vi "Step_Delay_Tommaso_equal_output.vi"() -> ()   [LabVIEW 2015]
uses:
  <vilib>/DAQmx/write.llb/DAQmx Write (Analog DBL 1Chan 1Samp).vi
  <vilib>/DAQmx/miscellaneous.llb/DAQmx Fill In Error Info.vi
  <vilib>/DAQmx/create/channels.llb/DAQmx Create Channel (AO-Voltage-Basic).vi
  <vilib>/Analysis/1siggen.llb/Ramp Pattern by Delta.vi
  subvi/Newport ESP301/Newport ESP301.lvlib
  <vilib>/Analysis/NI_AALBase.lvlib
panel:
  in  "Output_Steps":bool caption="Output steps?"
  in  "Dwell_positions":string[][](table)=[["-500", "3000"], ["-100", "3000"], ["0", "5000"], ["100", "5000"], ["500", "5000"], ["750", "10000"], ["1000", "10000"], ["", ""]]
  in  "Enable2":bool caption="Enable?"
  in  "Wait time [ms]":u32=1000 caption="Values <50 \nwon't work"
  out "StepSize [mm]":dbl=0.14989622900000002
  in  "stop 2":bool
  in  "StepSize [fs]":i32=1000
  in  "Enable?":bool
  out "a":waveform(dbl)(graph)={"t0"=timestamp(3629703941.150015 s since 1904-01-01), "dt"=1.0, "Y"=[-1.00695]}
  out "Waveform Chart":dbl(graph)=5.25341140860948
  out "x*y":dbl=0.9998993703837595
  in  "physical channels":tag="Dev3/ao1"
  out "DAC error":errorcluster
  out "ESP error":errorcluster
  out "run?":bool
  in  "set_vel":bool
  in  "velocity [fs/s]":dbl=333.564095198152
  in  "vel_mm":dbl=0.05 caption="velocity [mm/s]"
  out "meas. velocity":dbl
  in  "stop":bool
  out "output voltage":dbl=0.9998993703837595
  in  "start":bool
  in  "go2p1":bool
  out "position [mm]":dbl=-1.00695
  in  "p2 [mm]":dbl=-0.707153771
  in  "p1 [mm]":dbl=-1.006946229
  in  "interpolate output":bool
  in  "Delta2 [fs]":dbl=999.9999999999999
  in  "Delta1 [fs]":dbl=-999.9999999999999
  in  "Reference [mm]":dbl=-0.85705
  in  "Axis (1)":i32=3 min=1 max=3
  in  "Serial Link (RS232)":enum16{"RS232", "USB"}(ring)
  in  "VISA resource name":refnum<visa-resource-name>="COM9"
  in  "main_close":bool
  # "Interface panel"
  # "Velocity panel"
  # "Positions panel"
  # "Equally spaced steps panel"
  # "Controls panel"
  # "User-defined steps panel"
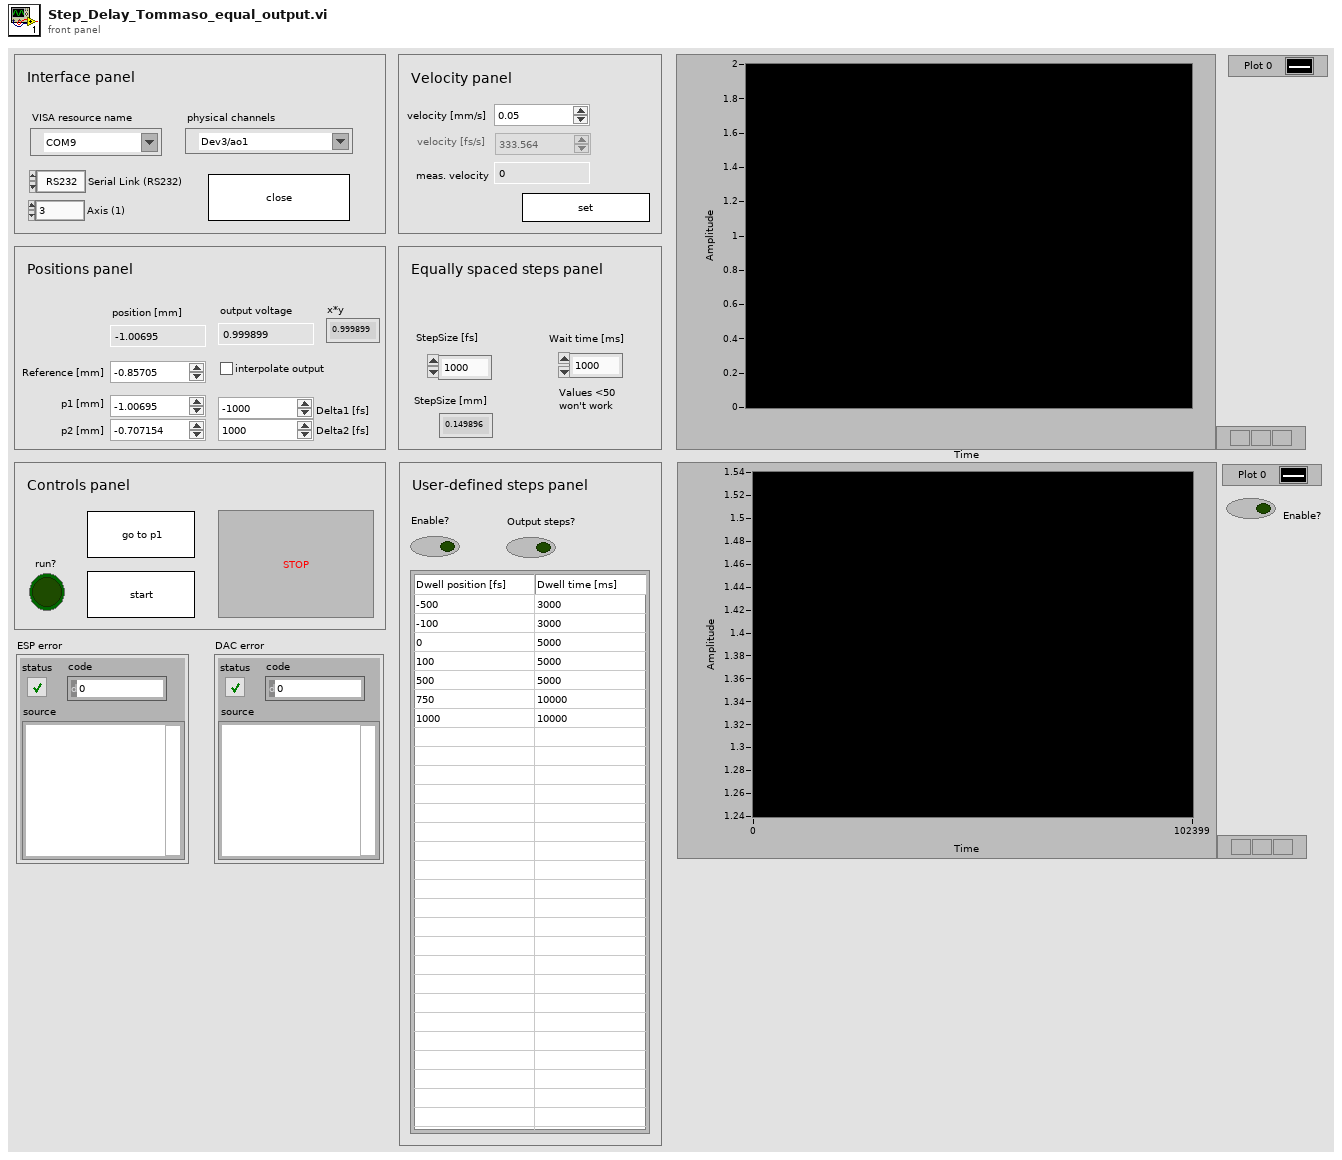
[diagram p1: front panel]
types:
  T1 = cluster{"dev1_data":refnum<queue>, "dev2_data":refnum<queue>}
  T2 = cluster{"dev1_cmd":refnum<queue>, "dev2_cmd":refnum<queue>}
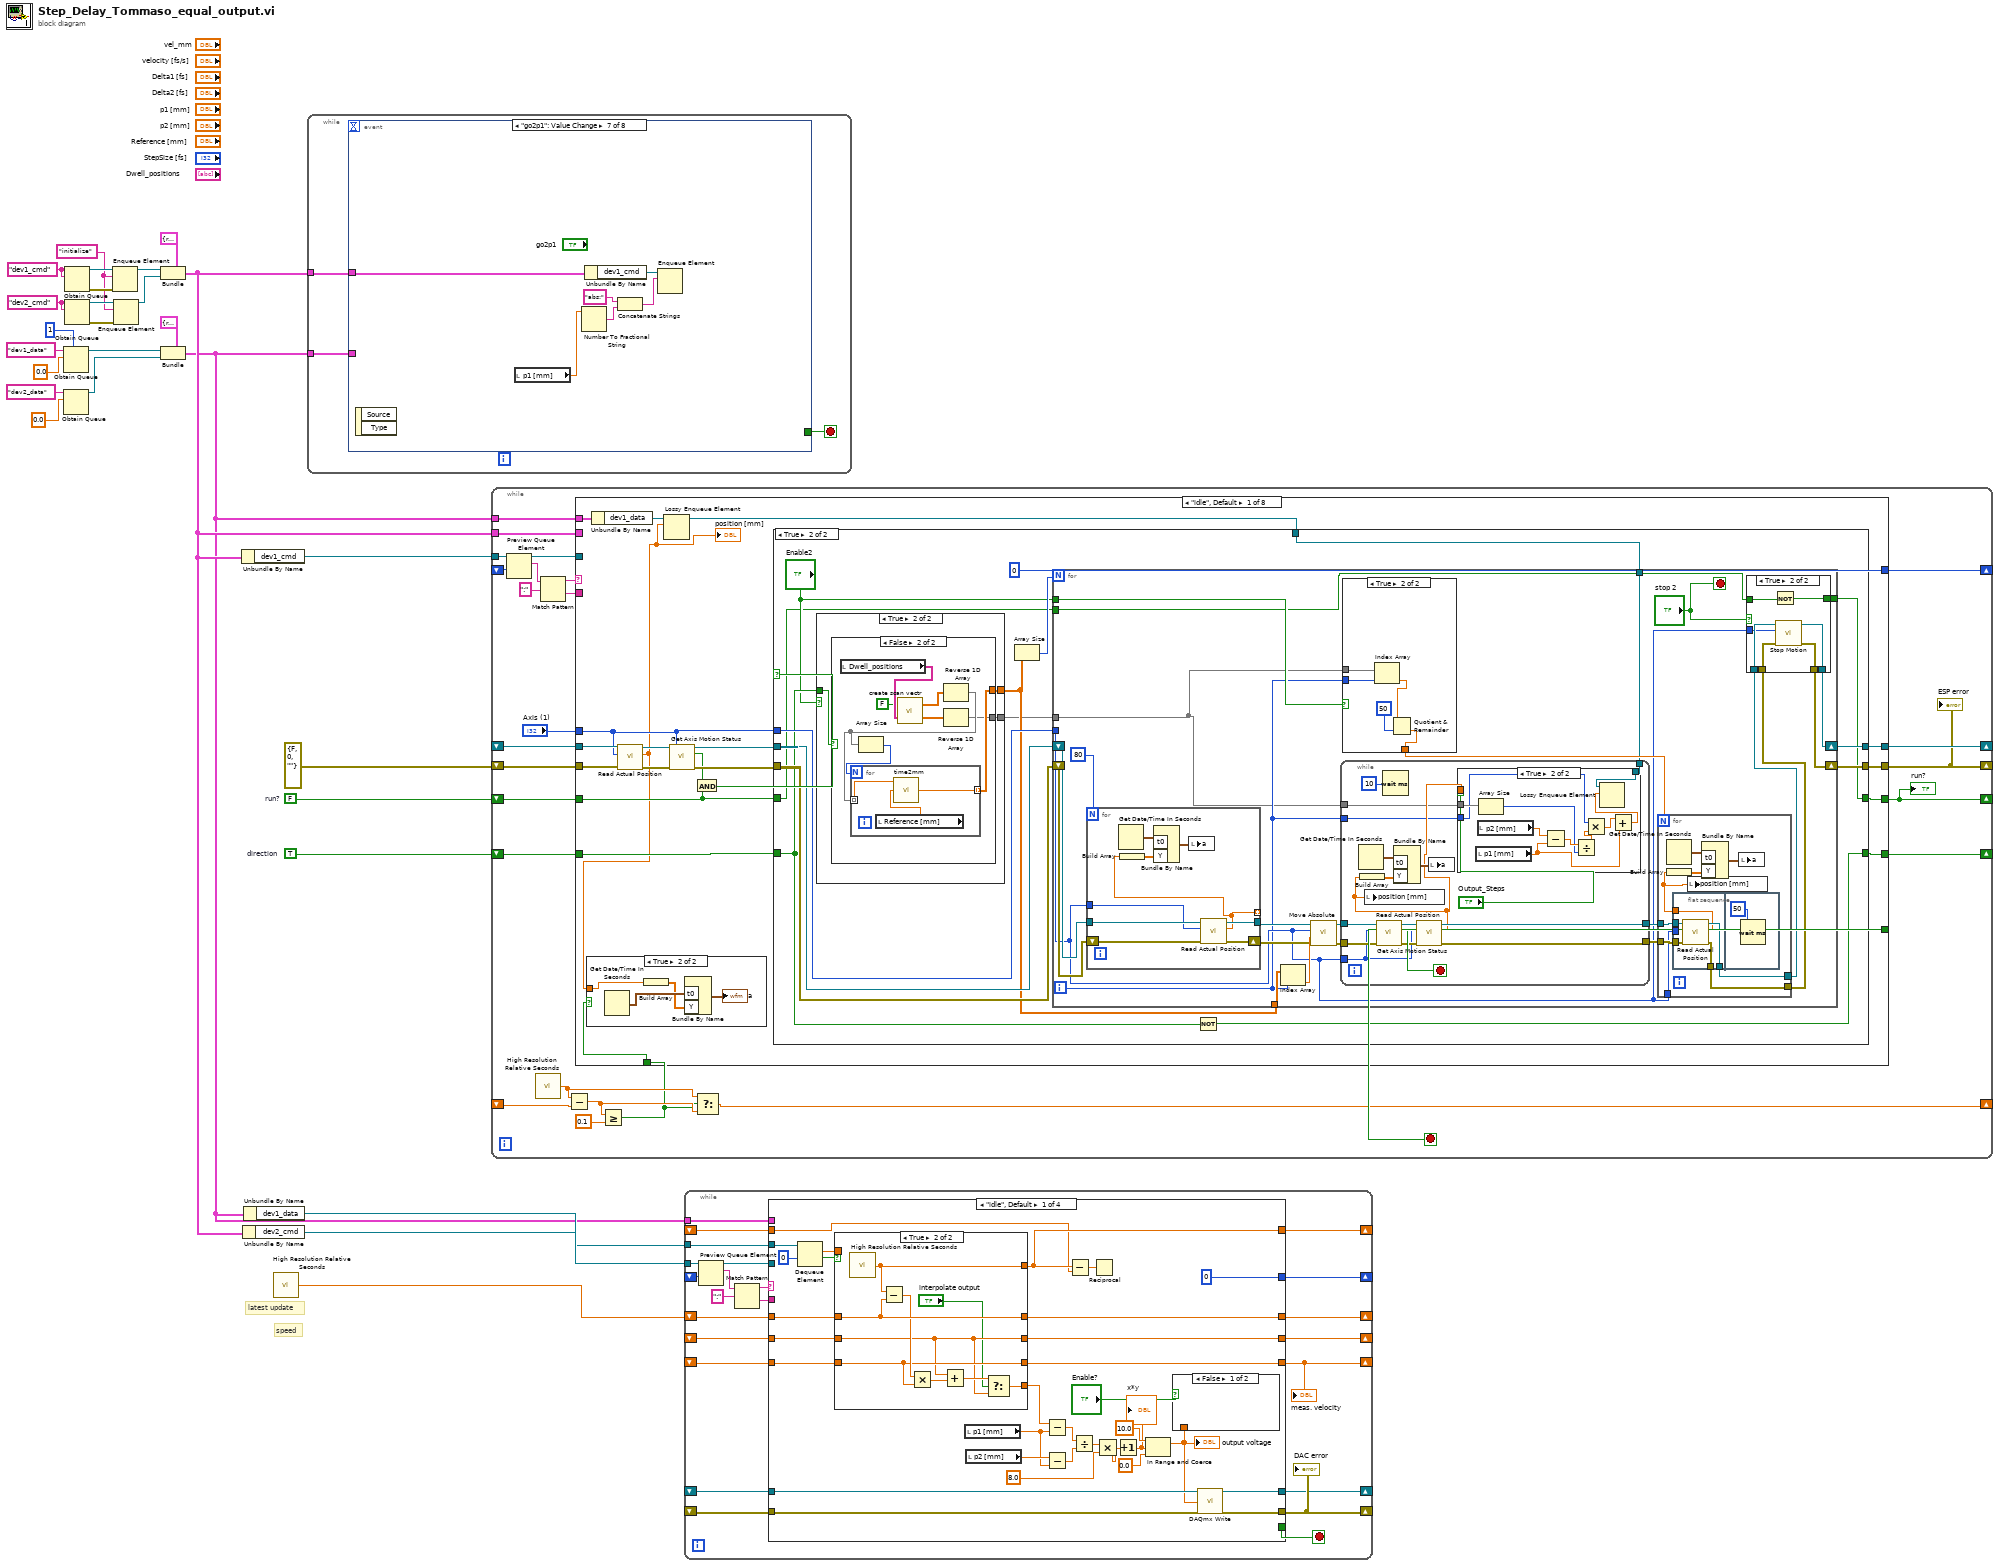
[diagram p0: block diagram]
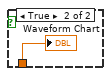
[diagram p2: hidden frame]
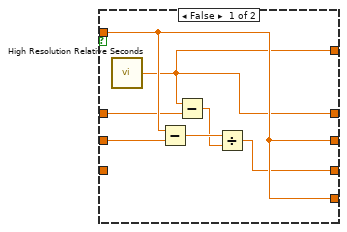
[diagram p3: hidden frame]
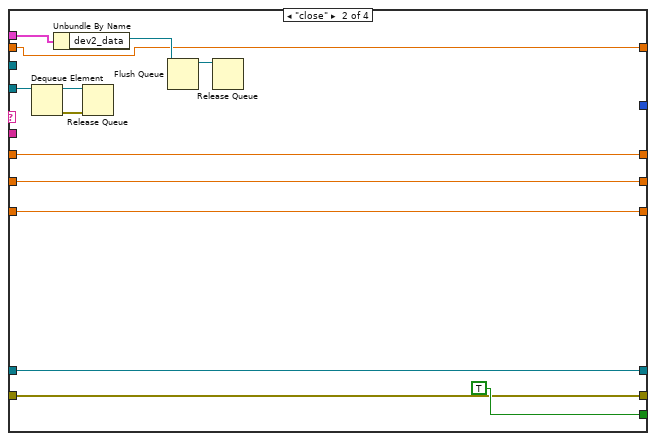
[diagram p4: hidden frame]
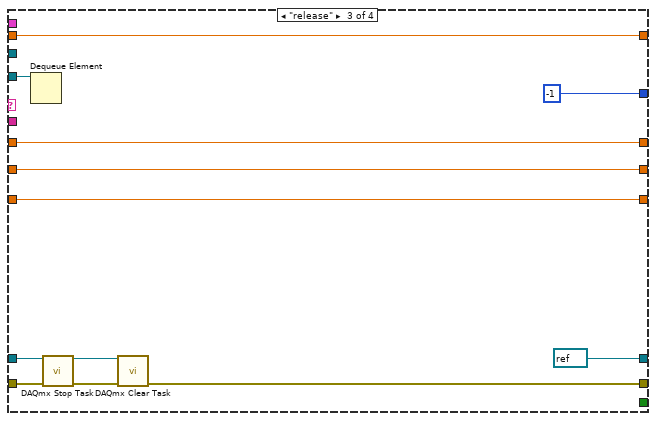
[diagram p5: hidden frame]
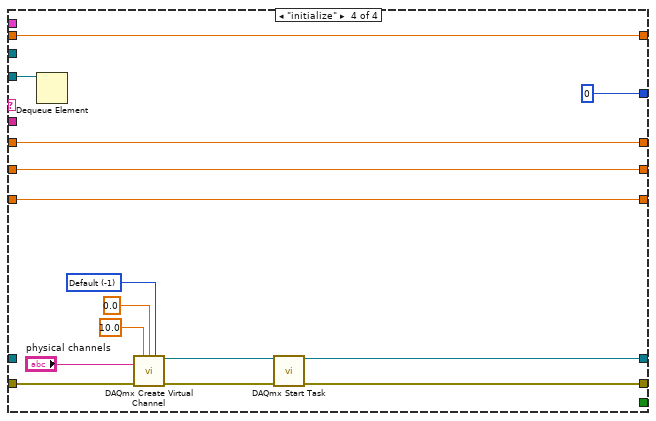
[diagram p6: hidden frame]
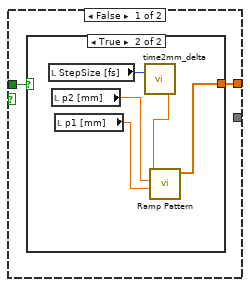
[diagram p9: hidden frame]
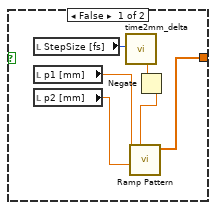
[diagram p10: hidden frame]
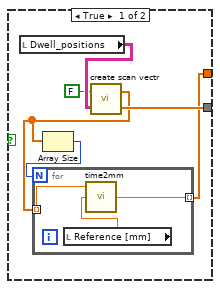
[diagram p11: hidden frame]
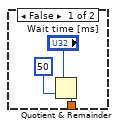
[diagram p13: hidden frame]
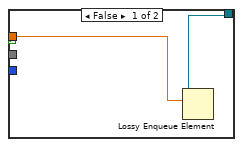
[diagram p14: hidden frame]
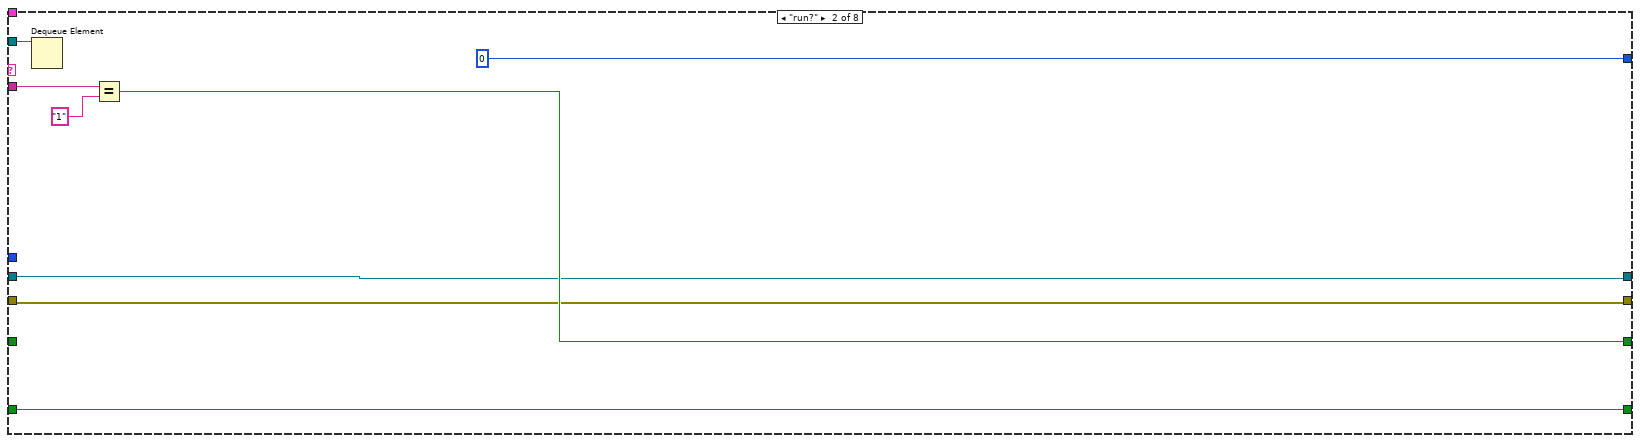
[diagram p15: hidden frame]
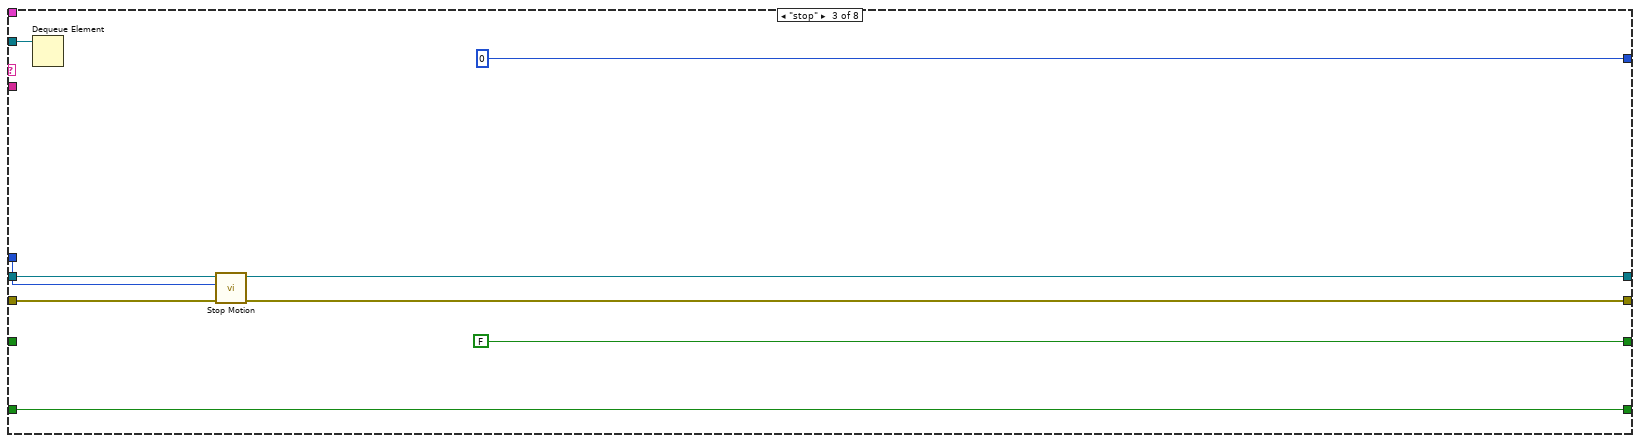
[diagram p16: hidden frame]
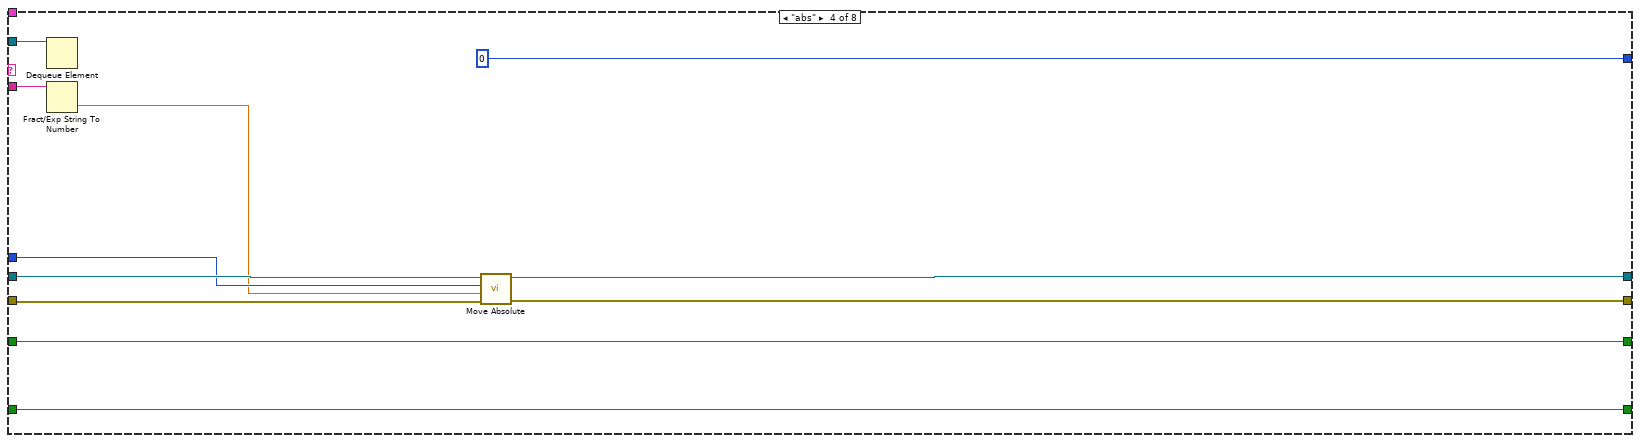
[diagram p17: hidden frame]
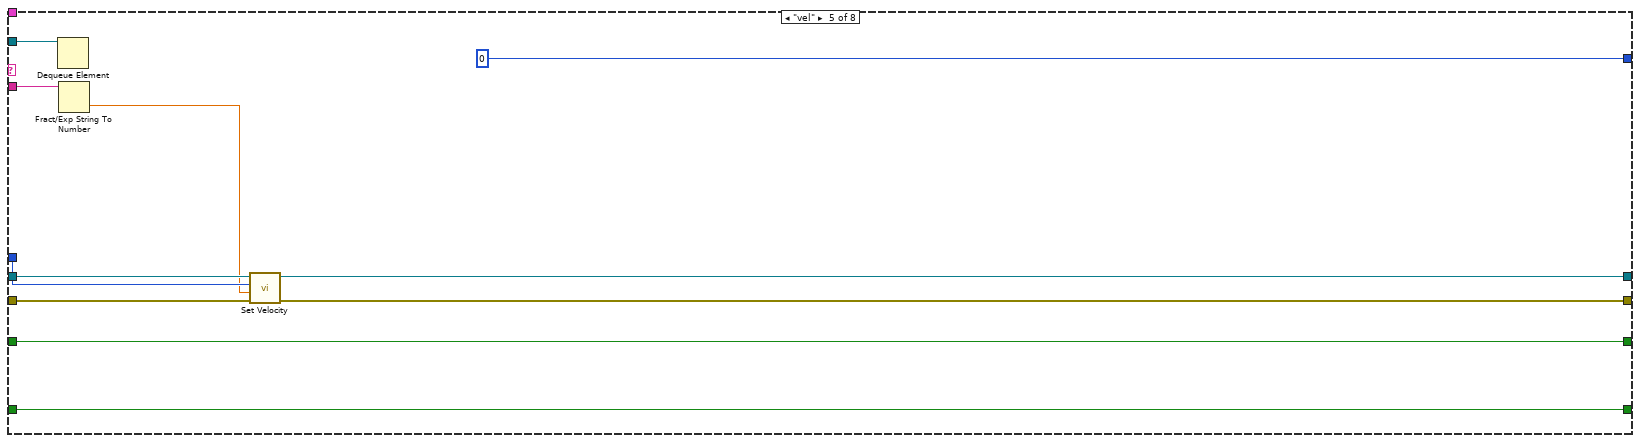
[diagram p18: hidden frame]
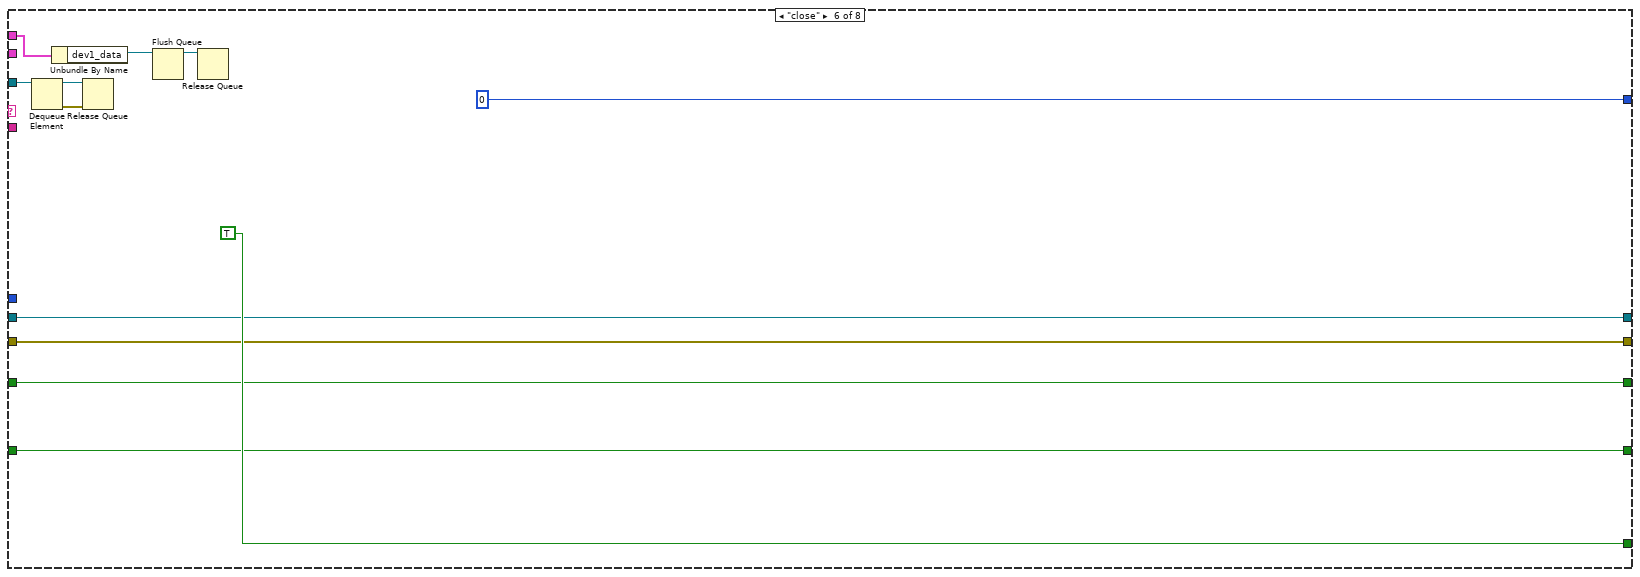
[diagram p19: hidden frame]
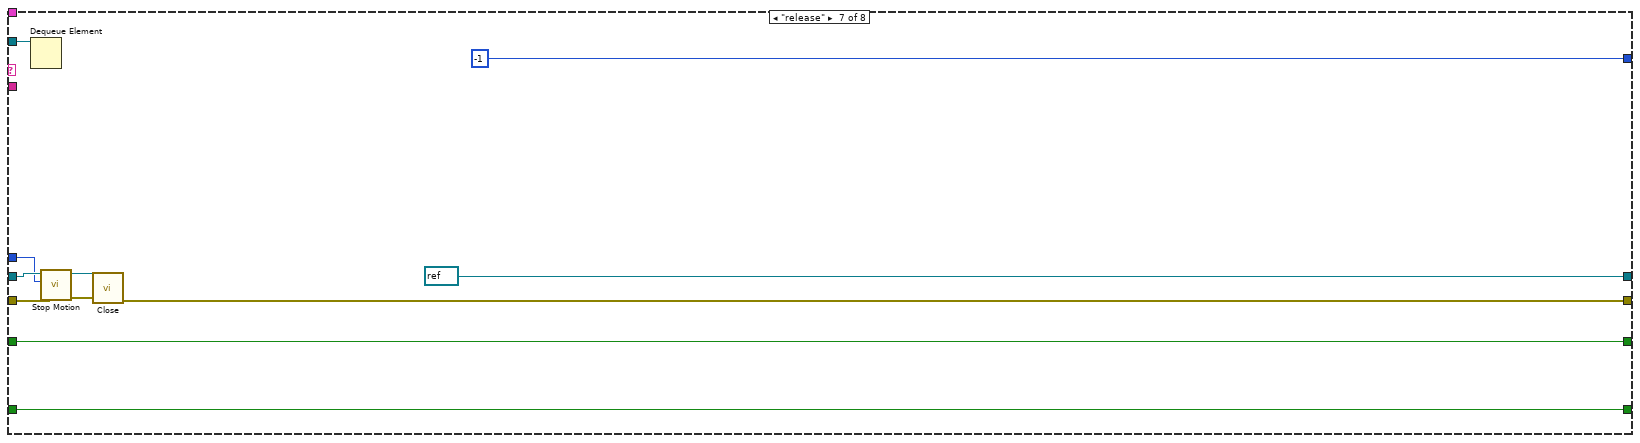
[diagram p20: hidden frame]
diagram:
  w1 = TRUE  # direction
  w4 = FALSE  # run?
  w15 = "dev2_cmd" ("name (unnamed)")
  w21 = "initialize" ("element")
  w16 = "dev1_cmd" ("name (unnamed)")
  # "speed"
  # "latest update"
  n1 = Obtain Queue(max queue size (-1, unlimited)=1, name (unnamed)="dev1_data", element data type=0.0) -> (queue out=w12:refnum<queue>)  [unwired: 2 in, 2 out]
  n2 = Obtain Queue(name (unnamed)="dev2_data", element data type=0.0) -> (queue out=w11:refnum<queue>)  [unwired: 3 in, 2 out]
  n3 = Obtain Queue(name (unnamed)=w16, element data type=w16) -> (queue out=w27:refnum<queue>, error out=w26:errorcluster)  [unwired: 3 in, 1 out]
  n4 = Obtain Queue(name (unnamed)=w15, element data type=w15) -> (queue out=w22:refnum<queue>, error out=w23:errorcluster)  [unwired: 3 in, 1 out]
  n5 = Enqueue Element(queue=w27, element=w21, error in (no error)=w26) -> (queue out=w24:refnum<queue>)  [unwired: 1 in, 2 out]
  n6 = Enqueue Element(queue=w22, element=w21, error in (no error)=w23) -> (queue out=w20:refnum<queue>)  [unwired: 1 in, 2 out]
  n7 = Bundle(cluster=T2 {"dev1_cmd"=refnum, "dev2_cmd"=refnum}, "dev1_cmd"=w24, "dev2_cmd"=w20) -> (w8:T2)
  n8 = Bundle(cluster=T1 {"dev1_data"=refnum, "dev2_data"=refnum}, "dev1_data"=w12, "dev2_data"=w11) -> (w2:T1)
  n9 = Unbundle By Name(w8) -> ("dev1_cmd"=w17:refnum<queue>)
  n10 = Unbundle By Name(w8) -> ("dev2_cmd"=w7:refnum<queue>)
  n11 = Unbundle By Name(w2) -> ("dev1_data"=w6:refnum<queue>)
  n12 = call <vilib>:"High Resolution Relative Seconds.vi"() -> ("relative seconds"=w5:dbl)
  n13 = while {
    tunnel: w8 -> [w30]
    tunnel: w2 -> [w29]
    stop <- w28 stop-if-true
    n14 = event shown="[6] \"go2p1\": Value Change" {
      selector: _ -> [_ _ _ _ _ _ _ _]
      dyn-events: _ -> [_ _ _ _ _ _ _ _]
      timeout: _ -> [_ _ _ _ _ _ _ _]
      tunnel: w30 -> [_ w34 _ _ w46 _ w64 w67]
      tunnel: w29 -> [_ _ _ _ _ _ _ _]
      tunnel: [_ _ _ _ _ _ _ TRUE] -> w28
      event Timeout {
        n15 = event-data() -> ()  [unwired: 1 in, 1 out]
      }
      event "start", "stop": Value Change {
        n16 = event-data() -> ()  [unwired: 1 in, 1 out]
        n17 = Boolean To (0,1)(Boolean="start") -> (0, 1=w32:i16)
        n18 = Number To Decimal String(number=w32) -> (decimal integer string=w31:string)  [unwired: 1 in]
        n19 = Unbundle By Name(w34) -> ("dev1_cmd"=w37:refnum<queue>)
        n20 = Concatenate Strings("run?:" ("string"), w31) -> (w36:string)
        n21 = Enqueue Element(queue=w37, element=w36) -> ()  [unwired: 2 in, 3 out]
      }
      event "StepSize [fs]": Value Change {
        n22 = event-data() -> ("NewVal"=w38:i32)  [unwired: 1 in, 5 out]
        n23 = call "time2mm_delta.vi"("Delta time"=w38) -> ("Delta position (mm)"=→"StepSize [mm]":dbl)  [unwired: 2 in]
      }
      event "Delta1 [fs]", "Delta2 [fs]": Value Change {
        n24 = event-data() -> ()  [unwired: 1 in, 1 out]
        n25 = local read "Reference [mm]"() -> (w41:dbl)
        n26 = local read "Delta2 [fs]"() -> (w42:dbl)
        n27 = local read "Delta1 [fs]"() -> (w44:dbl)
        n28 = call "time2mm.vi"("Offset (mm)"=w41, "time"=w44) -> ("position (mm)"=w43:dbl)  [unwired: 1 in]
        n29 = call "time2mm.vi"("Offset (mm)"=w41, "time"=w42) -> ("position (mm)"=w40:dbl)  [unwired: 1 in]
        n30 = local write "p2 [mm]"(w40) -> ()
        n31 = local write "p1 [mm]"(w43) -> ()
      }
      event "set_vel": Value Change {
        n32 = event-data() -> ()  [unwired: 1 in, 2 out]
        n33 = local read "vel_mm"() -> (w45:dbl)
        n34 = Number To Fractional String(number=w45) -> (F-format string=w49:string)  [unwired: 3 in]
        n35 = Unbundle By Name(w46) -> ("dev1_cmd"=w50:refnum<queue>)
        n36 = Concatenate Strings("vel:" ("string"), w49) -> (w48:string)
        n37 = Enqueue Element(queue=w50, element=w48) -> ()  [unwired: 2 in, 3 out]
      }
      event "p1 [mm]", "p2 [mm]", "Reference [mm]", "vel_mm": Value Change {
        n38 = event-data() -> ()  [unwired: 1 in, 2 out]
        n39 = local read "Reference [mm]"() -> (w56:dbl)
        n40 = local read "vel_mm"() -> (w53:dbl)
        n41 = local read "p1 [mm]"() -> (w57:dbl)
        n42 = local read "p2 [mm]"() -> (w58:dbl)
        n43 = call "mm2time.vi"("Offset (mm)"=0.0, "distance (mm)"=w53) -> ("time in fs"=w52:dbl)  [unwired: 1 in]
        n44 = call "mm2time.vi"("Offset (mm)"=w56, "distance (mm)"=w57) -> ("time in fs"=w54:dbl)  [unwired: 1 in]
        n45 = call "mm2time.vi"("Offset (mm)"=w56, "distance (mm)"=w58) -> ("time in fs"=w55:dbl)  [unwired: 1 in]
        n46 = local write "velocity [fs/s]"(w52) -> ()
        n47 = local write "Delta1 [fs]"(w54) -> ()
        n48 = local write "Delta2 [fs]"(w55) -> ()
      }
      event "go2p1": Value Change {
        n49 = event-data() -> ()  [unwired: 1 in, 2 out]
        n50 = local read "p1 [mm]"() -> (w59:dbl)
        n51 = Number To Fractional String(number=w59) -> (F-format string=w62:string)  [unwired: 3 in]
        n52 = Unbundle By Name(w64) -> ("dev1_cmd"=w63:refnum<queue>)
        n53 = Concatenate Strings("abs:" ("string"), w62) -> (w60:string)
        n54 = Enqueue Element(queue=w63, element=w60) -> ()  [unwired: 2 in, 3 out]
      }
      event "main_close": Value Change {
        n55 = event-data() -> ()  [unwired: 1 in, 1 out]
        n56 = Cluster To Array(cluster=w67) -> (array=w66:refnum<queue>[])
        n57 = for {
          tunnel: w66 -> [w72] mode=indexing
          n58 = Flush Queue(queue=w72) -> (queue out=w68:refnum<queue>)  [unwired: 1 in, 2 out]
          n59 = Enqueue Element(queue=w68, element="release") -> (queue out=w70:refnum<queue>)  [unwired: 2 in, 2 out]
          n60 = Enqueue Element(queue=w70, element="close") -> ()  [unwired: 2 in, 3 out]
        }
      }
    }
  }
  n61 = while {
    tunnel: w8 -> [w93]
    tunnel: w17 -> [w98]
    tunnel: w2 -> [w90]
    shift-right: [w88] -> _
    shift-left: _ -> [w89]
    shift-right: [w87] -> _
    shift-left: _ -> [w84]
    shift-right: [w86] -> _
    shift-left: errorcluster {"status"=FALSE, "code"=0, "source"=""} ("error out") -> [w85]
    shift-right: [w81] -> _
    shift-left: w4 -> [w82]
    shift-right: [w79] -> _
    shift-left: w1 -> [w80]
    shift-right: [w73] -> _
    shift-left: _ -> [w78]
    stop <- w91 stop-if-true
    n62 = Preview Queue Element(queue=w98, timeout in ms (-1)=w89) -> (queue out=w92:refnum<queue>, element=w97:string)  [unwired: 1 in, 2 out]
    n63 = call <vilib>:"High Resolution Relative Seconds.vi"() -> ("relative seconds"=w75:dbl)
    n64 = Match Pattern(string=w97, regular expression=":") -> (before substring=w95:string, after substring=w94:string)  [unwired: 1 in, 2 out]
    n65 = Subtract(x=w75, y=w78) -> (x-y=w76:dbl)
    n66 = Greater Or Equal?(x=w76, y=0.1) -> (x >= y?=w74:bool)
    n67 = case shown="\"idle\", Default" w95 {
      tunnel: w94 -> [_ w281 _ w300 w307 _ _ _]
      tunnel: w93 -> [_ _ _ _ _ _ _ _]
      tunnel: w92 -> [_ w279 w283 w301 w305 w324 w334 w344]
      tunnel: [_ _ _ _ _ TRUE _ _] -> w91
      tunnel: w90 -> [w118 _ _ _ _ w316 _ _]
      tunnel: [0 0 0 0 0 0 -1 0] -> w88
      tunnel: [w116 w274 w288 w297 w312 w320 refnum<visa-resource-name> refnum ("VISA resource name out") w340] -> w87
      tunnel: [w115 w275 w287 w296 w311 w319 w333 w339] -> w86
      tunnel: w85 -> [w113 w275 w289 w298 w310 w319 w329 _]
      tunnel: w84 -> [w114 w274 w290 w299 w309 w320 w326 _]
      tunnel: "Axis (1)" -> [w104 _ w286 w295 w308 _ w325 w341]
      tunnel: w82 -> [w102 _ _ w292 w303 w317 w331 w345]
      tunnel: [w110 w277 FALSE ("run?") w292 w303 w317 w331 w345] -> w81
      tunnel: w80 -> [w111 w276 w282 w291 w302 w313 w330 w336]
      tunnel: [w112 w276 w282 w291 w302 w313 w330 w336] -> w79
      tunnel: w74 -> [w99 _ _ _ _ _ _ _]
      frame "idle", Default {
        n68 = Unbundle By Name(w118) -> ("dev1_data"=w117:refnum<queue>)
        n69 = call "Read Actual Position.vi"("error in (no error)"=w113, "Axis (1)"=w104, "VISA resource name"=w114) -> ("error out"=w107:errorcluster, "Position (units)"=w100:dbl, "VISA resource name out"=w108:refnum<visa-resource-name>)  [unwired: 2 in]
        "position [mm]" <- w100
        n70 = case shown="True" w99 {
          tunnel: w100 -> [_ w123]
          frame False {
          }
          frame True {
            n71 = Get Date/Time In Seconds() -> (seconds since 1Jan1904=w122:timestamp)
            n72 = Build Array(w123) -> (w121:dbl[])
            n73 = Bundle By Name("t0"=w122, "Y"=w121) -> (→"a":waveform(dbl))  [unwired: 1 in]
          }
        }
        n74 = Lossy Enqueue Element(queue=w117, element=w100) -> (queue out=w109:refnum<queue>)  [unwired: 1 in, 3 out]
        n75 = call "Get Axis Motion Status.vi"("error in (no error)"=w107, "Axis (1)"=w104, "VISA resource name"=w108) -> ("error out"=w105:errorcluster, "Motion Done"=w103:bool, "VISA resource name out"=w106:refnum<visa-resource-name>)  [unwired: 2 in]
        n76 = And(x=w103, y=w102) -> (x .and. y?=w101:bool)
        n77 = case shown="True" w101 {
          tunnel: w106 -> [w127 w140]
          tunnel: w105 -> [w126 w141]
          tunnel: [w127 w139] -> w116
          tunnel: [w126 w138] -> w115
          tunnel: w104 -> [_ w137]
          tunnel: [w125 w136] -> w112
          tunnel: w111 -> [w125 w135]
          tunnel: w102 -> [w124 w130]
          tunnel: [w124 w129] -> w110
          tunnel: w109 -> [_ w128]
          frame False {
          }
          frame True {
            n78 = case shown="True" "Enable2" {
              tunnel: w135 -> [w143 w155]
              tunnel: [w142 w156] -> w134
              tunnel: [_ w157] -> w131
              frame False {
                n79 = case shown="True" w143 {
                  tunnel: [w147 w152] -> w142
                  frame False {
                    n80 = local read "StepSize [fs]"() -> (w144:i32)
                    n81 = local read "p1 [mm]"() -> (w149:dbl)
                    n82 = local read "p2 [mm]"() -> (w148:dbl)
                    n83 = call "time2mm_delta.vi"("Delta time"=w144) -> ("Delta position (mm)"=w145:dbl)  [unwired: 2 in]
                    n84 = Negate(x=w145) -> (-x=w146:dbl)
                    n85 = call-poly <vilib>:"Ramp Pattern.vi"("start"=w148, "end"=w149, "delta"=w146) -> ("Ramp Pattern"=w147:dbl[])  [unwired: 6 in, 2 out]
                  }
                  frame True {
                    n86 = local read "StepSize [fs]"() -> (w150:i32)
                    n87 = local read "p2 [mm]"() -> (w153:dbl)
                    n88 = local read "p1 [mm]"() -> (w154:dbl)
                    n89 = call "time2mm_delta.vi"("Delta time"=w150) -> ("Delta position (mm)"=w151:dbl)  [unwired: 2 in]
                    n90 = call-poly <vilib>:"Ramp Pattern.vi"("start"=w154, "end"=w153, "delta"=w151) -> ("Ramp Pattern"=w152:dbl[])  [unwired: 6 in, 2 out]
                  }
                }
              }
              frame True {
                n91 = case shown="False" w155 {
                  tunnel: [w161 w167] -> w157
                  tunnel: [w160 w172] -> w156
                  frame True {
                    n92 = local read "Dwell_positions"() -> (w163:string[][])
                    n93 = call "create scan vectr.vi"("Table Control"=w163, "waypoint mode?"=FALSE) -> ("Array 2"=w161:dbl[], "Array"=w159:dbl[])
                    n94 = Array Size(array=w159) -> (size(s)=w158:i32)
                    n95 = for {
                      N: w158 -> [_]
                      tunnel: w159 -> [w166] mode=indexing
                      tunnel: [w165] -> w160 mode=indexing
                      n96 = local read "Reference [mm]"() -> (w164:dbl)
                      n97 = call "time2mm.vi"("Offset (mm)"=w164, "time"=w166) -> ("position (mm)"=w165:dbl)  [unwired: 1 in]
                    }
                  }
                  frame False {
                    n98 = local read "Dwell_positions"() -> (w174:string[][])
                    n99 = call "create scan vectr.vi"("Table Control"=w174, "waypoint mode?"=FALSE) -> ("Array 2"=w168:dbl[], "Array"=w169:dbl[])
                    n100 = Reverse 1D Array(array=w169) -> (reversed array=w170:dbl[])
                    n101 = Array Size(array=w170) -> (size(s)=w171:i32)
                    n102 = for {
                      N: w171 -> [_]
                      tunnel: w170 -> [w177] mode=indexing
                      tunnel: [w176] -> w172 mode=indexing
                      n103 = local read "Reference [mm]"() -> (w175:dbl)
                      n104 = call "time2mm.vi"("Offset (mm)"=w175, "time"=w177) -> ("position (mm)"=w176:dbl)  [unwired: 1 in]
                    }
                    n105 = Reverse 1D Array(array=w168) -> (reversed array=w167:dbl[])
                  }
                }
              }
            }
            n106 = Array Size(array=w134) -> (size(s)=w133:i32)
            n107 = for {
              N: w133 -> [_]
              tunnel: w137 -> [w183]
              tunnel: w134 -> [w196]
              shift-right: [w185] -> w138
              shift-left: w141 -> [w200]
              shift-right: [w187] -> w139
              shift-left: w140 -> [w199]
              tunnel: "Enable2" -> [w189]
              tunnel: w131 -> [w178]
              tunnel: w130 -> [w182]
              tunnel: [w181] -> w129
              tunnel: w128 -> [w180]
              i -> [w179]
              stop <- "stop 2" stop-if-true
              n108 = for {
                N: 80 -> [_]
                tunnel: w199 -> [w273]
                tunnel: [w272] -> w198
                shift-right: [w269] -> w193
                shift-left: w200 -> [w271]
                tunnel: w183 -> [w270]
                tunnel: [w266] -> _ mode=indexing
                n109 = Get Date/Time In Seconds() -> (seconds since 1Jan1904=w267:timestamp)
                n110 = call "Read Actual Position.vi"("error in (no error)"=w271, "Axis (1)"=w270, "VISA resource name"=w273) -> ("error out"=w269:errorcluster, "Position (units)"=w266:dbl, "VISA resource name out"=w272:refnum<visa-resource-name>)  [unwired: 2 in]
                n111 = Build Array(w266) -> (w268:dbl[])
                n112 = Bundle By Name("t0"=w267, "Y"=w268) -> (w265:waveform(dbl))  [unwired: 1 in]
                n113 = local write "a"(w265) -> ()
              }
              n114 = Index Array(array=w196, index=w179) -> (element=w197:dbl)
              n115 = call "Move Absolute.vi"("error in (no error)"=w193, "Position (0 units)"=w197, "Axis (1)"=w183, "VISA resource name"=w198) -> ("error out"=w194:errorcluster, "VISA resource name out"=w195:refnum<visa-resource-name>)  [unwired: 2 in]
              n116 = while {
                tunnel: w195 -> [w252]
                tunnel: [w247] -> w190
                tunnel: w194 -> [w251]
                tunnel: [w245] -> w191
                tunnel: w183 -> [w244]
                tunnel: w180 -> [w239]
                tunnel: w179 -> [w237]
                tunnel: w178 -> [w236]
                stop <- w249 stop-if-true
                n117 = Get Date/Time In Seconds() -> (seconds since 1Jan1904=w243:timestamp)
                n118 = call "Get Axis Motion Status.vi"("error in (no error)"=w251, "Axis (1)"=w244, "VISA resource name"=w252) -> ("error out"=w246:errorcluster, "Motion Done"=w249:bool, "VISA resource name out"=w248:refnum<visa-resource-name>)  [unwired: 2 in]
                n119 = Wait (ms)(milliseconds to wait=10) -> ()  [unwired: 1 out]
                n120 = call "Read Actual Position.vi"("error in (no error)"=w246, "Axis (1)"=w244, "VISA resource name"=w248) -> ("error out"=w245:errorcluster, "Position (units)"=w240:dbl, "VISA resource name out"=w247:refnum<visa-resource-name>)  [unwired: 2 in]
                n121 = Build Array(w240) -> (w242:dbl[])
                n122 = local write "position [mm]"(w240) -> ()
                n123 = Bundle By Name("t0"=w243, "Y"=w242) -> (w241:waveform(dbl))  [unwired: 1 in]
                n124 = local write "a"(w241) -> ()
                n125 = case shown="True" "Output_Steps" {
                  tunnel: w240 -> [w254 _]
                  tunnel: w239 -> [w253 w259]
                  tunnel: w237 -> [_ w255]
                  tunnel: w236 -> [_ w262]
                  frame False {
                    n126 = Lossy Enqueue Element(queue=w253, element=w254) -> ()  [unwired: 1 in, 4 out]
                  }
                  frame True {
                    n127 = local read "p1 [mm]"() -> (w258:dbl)
                    n128 = local read "p2 [mm]"() -> (w264:dbl)
                    n129 = Array Size(array=w262) -> (size(s)=w261:i32)
                    n130 = Subtract(x=w264, y=w258) -> (x-y=w263:dbl)
                    n131 = Divide(x=w263, y=w261) -> (x/y=w260:dbl)
                    n132 = Multiply(x=w255, y=w260) -> (x*y=w257:dbl)
                    n133 = Add(x=w257, y=w258) -> (x+y=w256:dbl)
                    n134 = Lossy Enqueue Element(queue=w259, element=w256) -> ()  [unwired: 1 in, 4 out]
                  }
                }
              }
              n135 = case shown="True" w189 {
                tunnel: [w212 w218] -> w192
                tunnel: w179 -> [_ w216]
                tunnel: w178 -> [_ w215]
                frame False {
                  n136 = Quotient & Remainder(x="Wait time [ms]", y=50) -> (floor(x/y)=w212:u32)  [unwired: 1 out]
                }
                frame True {
                  n137 = Index Array(array=w215, index=w216) -> (element=w217:dbl)
                  n138 = Quotient & Remainder(x=w217, y=50) -> (floor(x/y)=w218:dbl)  [unwired: 1 out]
                }
              }
              n139 = for {
                N: w192 -> [_]
                tunnel: w191 -> [w228]
                tunnel: [w227] -> w186
                tunnel: w190 -> [w226]
                tunnel: [w225] -> w188
                tunnel: w183 -> [w224]
                n140 = Get Date/Time In Seconds() -> (seconds since 1Jan1904=w222:timestamp)
                n141 = Build Array(w220) -> (w223:dbl[])
                n142 = flat-sequence {
                  tunnel: w228 -> [w234]
                  tunnel: [w233] -> w227
                  tunnel: w226 -> [w232]
                  tunnel: [w231] -> w225
                  tunnel: w224 -> [w230]
                  tunnel: [w229] -> w220
                  frame #0 {
                    n143 = call "Read Actual Position.vi"("error in (no error)"=w234, "Axis (1)"=w230, "VISA resource name"=w232) -> ("error out"=w233:errorcluster, "Position (units)"=w229:dbl, "VISA resource name out"=w231:refnum<visa-resource-name>)  [unwired: 2 in]
                  }
                  frame #1 {
                    n144 = Wait (ms)(milliseconds to wait=50) -> ()  [unwired: 1 out]
                  }
                }
                n145 = local write "position [mm]"(w220) -> ()
                n146 = Bundle By Name("t0"=w222, "Y"=w223) -> (w221:waveform(dbl))  [unwired: 1 in]
                n147 = local write "a"(w221) -> ()
              }
              n148 = case shown="True" "stop 2" {
                tunnel: w188 -> [w204 w211]
                tunnel: [w204 w210] -> w187
                tunnel: w186 -> [w203 w209]
                tunnel: [w203 w208] -> w185
                tunnel: w183 -> [_ w207]
                tunnel: w182 -> [w202 w206]
                tunnel: [w202 w205] -> w181
                frame False {
                }
                frame True {
                  n149 = Not(x=w206) -> (.not. x?=w205:bool)
                  n150 = call "Stop Motion.vi"("error in (no error)"=w209, "Axis (1)"=w207, "VISA resource name"=w211) -> ("error out"=w208:errorcluster, "VISA resource name out"=w210:refnum<visa-resource-name>)  [unwired: 3 in]
                }
              }
            }
            n151 = Not(x=w135) -> (.not. x?=w136:bool)
          }
        }
      }
      frame "run?" {
        n152 = Dequeue Element(queue=w279) -> ()  [unwired: 2 in, 4 out]
        n153 = Equal?(x=w281, y="1") -> (x = y?=w277:bool)
      }
      frame "stop" {
        n154 = Dequeue Element(queue=w283) -> ()  [unwired: 2 in, 4 out]
        n155 = call "Stop Motion.vi"("error in (no error)"=w289, "Axis (1)"=w286, "VISA resource name"=w290) -> ("error out"=w287:errorcluster, "VISA resource name out"=w288:refnum<visa-resource-name>)  [unwired: 3 in]
      }
      frame "abs" {
        n156 = Dequeue Element(queue=w301) -> ()  [unwired: 2 in, 4 out]
        n157 = Fract/Exp String To Number(string=w300) -> (number=w294:dbl)  [unwired: 3 in, 1 out]
        n158 = call "Move Absolute.vi"("error in (no error)"=w298, "Position (0 units)"=w294, "Axis (1)"=w295, "VISA resource name"=w299) -> ("error out"=w296:errorcluster, "VISA resource name out"=w297:refnum<visa-resource-name>)  [unwired: 2 in]
      }
      frame "vel" {
        n159 = Dequeue Element(queue=w305) -> ()  [unwired: 2 in, 4 out]
        n160 = Fract/Exp String To Number(string=w307) -> (number=w306:dbl)  [unwired: 3 in, 1 out]
        n161 = call "Set Velocity.vi"("error in (no error)"=w310, "Velocity (units/s)"=w306, "Axis (1)"=w308, "VISA resource name"=w309) -> ("error out"=w311:errorcluster, "VISA resource name out"=w312:refnum<visa-resource-name>)  [unwired: 2 in]
      }
      frame "close" {
        n162 = Dequeue Element(queue=w324) -> (queue out=w323:refnum<queue>, error out=w322:errorcluster)  [unwired: 2 in, 2 out]
        n163 = Unbundle By Name(w316) -> ("dev1_data"=w314:refnum<queue>)
        n164 = Release Queue(queue=w323, error in (no error)=w322) -> ()  [unwired: 1 in, 3 out]
        n165 = Flush Queue(queue=w314) -> (queue out=w315:refnum<queue>)  [unwired: 1 in, 2 out]
        n166 = Release Queue(queue=w315) -> ()  [unwired: 2 in, 3 out]
      }
      frame "release" {
        n167 = Dequeue Element(queue=w334) -> ()  [unwired: 2 in, 4 out]
        n168 = call "Stop Motion.vi"("error in (no error)"=w329, "Axis (1)"=w325, "VISA resource name"=w326) -> ("error out"=w328:errorcluster, "VISA resource name out"=w327:refnum<visa-resource-name>)  [unwired: 3 in]
        n169 = call "Close.vi"("error in (no error)"=w328, "VISA resource name"=w327) -> ("error out"=w333:errorcluster)  [unwired: 9 in]
      }
      frame "initialize" {
        n170 = Dequeue Element(queue=w344) -> ()  [unwired: 2 in, 4 out]
        n171 = call "Initialize.vi"("VISA resource name"="VISA resource name", "error in (no error)"=errorcluster {"status"=FALSE, "code"=0, "source"=""}, "Serial Link (RS232)"="Serial Link (RS232)") -> ("VISA resource name out"=w343:refnum<visa-resource-name>, "error out"=w342:errorcluster)  [unwired: 6 in]
        n172 = call "Get Velocity.vi"("error in (no error)"=w342, "Axis (1)"=w341, "VISA resource name"=w343) -> ("error out"=w339:errorcluster, "Velocity (units/s)"=w338:dbl, "VISA resource name out"=w340:refnum<visa-resource-name>)  [unwired: 2 in]
        n173 = local write "vel_mm"(w338) -> ()
      }
    }
    "run?" <- w81
    "ESP error" <- w86
    n174 = Select(t=w75, s=w74, f=w76) -> (s? t:f=w73:dbl)
  }
  n175 = while {
    shift-right: [w364] -> _
    shift-left: _ -> [w365]
    shift-right: [w363] -> _
    shift-left: _ -> [w362]
    tunnel: w7 -> [w361]
    shift-right: [w360] -> _
    shift-left: _ -> [w359]
    tunnel: w6 -> [w358]
    shift-right: [w357] -> _
    shift-left: _ -> [w354]
    shift-right: [w356] -> _
    shift-left: w5 -> [w355]
    shift-right: [w349] -> _
    shift-left: _ -> [w353]
    tunnel: w2 -> [w352]
    shift-right: [w351] -> _
    shift-left: _ -> [w350]
    stop <- w366 stop-if-true
    n176 = Preview Queue Element(queue=w361, timeout in ms (-1)=w365) -> (queue out=w367:refnum<queue>, element=w371:string)  [unwired: 1 in, 2 out]
    n177 = Match Pattern(string=w371, regular expression=":") -> (before substring=w369:string, after substring=w368:string)  [unwired: 1 in, 2 out]
    n178 = case shown="\"idle\", Default" w369 {
      tunnel: w368 -> [_ _ _ _]
      tunnel: w367 -> [_ w432 w443 w451]
      tunnel: [_ TRUE _ _] -> w366
      tunnel: [0 _ -1 0] -> w364
      tunnel: [w398 w428 w442 w452] -> w363
      tunnel: w362 -> [w396 w428 w439 w459]
      tunnel: [w399 w427 refnum<k21> refnum ("task out") w453] -> w360
      tunnel: w359 -> [w397 w427 w440 _]
      tunnel: w358 -> [w400 _ _ _]
      tunnel: [w394 w425 w435 w448] -> w357
      tunnel: [w393 w426 w436 w449] -> w356
      tunnel: w355 -> [w391 w426 w436 w449]
      tunnel: w354 -> [w392 w425 w435 w448]
      tunnel: [w390 w424 w434 w447] -> w349
      tunnel: w353 -> [w389 w424 w434 w447]
      tunnel: w352 -> [_ w421 _ _]
      tunnel: [w378 w420 w433 w445] -> w351
      tunnel: w350 -> [w377 w420 w433 w445]
      frame "idle", Default {
        n179 = Dequeue Element(queue=w400, timeout in ms (-1)=0) -> (element=w395:dbl, timed out?=w379:bool)  [unwired: 1 in, 2 out]
        n180 = case shown="True" w379 {
          tunnel: w395 -> [w410 _]
          tunnel: [w410 w412] -> w388
          tunnel: [w410 w414] -> w394
          tunnel: [w404 w419] -> w393
          tunnel: w392 -> [w409 w414]
          tunnel: w391 -> [w408 w419]
          tunnel: [w405 w416] -> w390
          tunnel: w389 -> [_ w416]
          tunnel: [w404 w411] -> w378
          frame False {
            n181 = call <vilib>:"High Resolution Relative Seconds.vi"() -> ("relative seconds"=w404:dbl)
            n182 = Subtract(x=w410, y=w409) -> (x-y=w407:dbl)
            n183 = Subtract(x=w404, y=w408) -> (x-y=w406:dbl)
            n184 = Divide(x=w407, y=w406) -> (x/y=w405:dbl)
          }
          frame True {
            n185 = call <vilib>:"High Resolution Relative Seconds.vi"() -> ("relative seconds"=w411:dbl)
            n186 = Subtract(x=w411, y=w419) -> (x-y=w418:dbl)
            n187 = Multiply(x=w418, y=w416) -> (x*y=w417:dbl)
            n188 = Add(x=w414, y=w417) -> (x+y=w415:dbl)
            n189 = Select(t=w415, s="interpolate output", f=w414) -> (s? t:f=w412:dbl)
          }
        }
        n190 = local read "p1 [mm]"() -> (w386:dbl)
        n191 = local read "p2 [mm]"() -> (w387:dbl)
        n192 = Subtract(x=w388, y=w386) -> (x-y=w385:dbl)
        n193 = Subtract(x=w387, y=w386) -> (x-y=w384:dbl)
        n194 = Subtract(x=w378, y=w377) -> (x-y=w376:dbl)
        n195 = Divide(x=w385, y=w384) -> (x/y=w383:dbl)
        n196 = Reciprocal(x=w376) -> ()  [unwired: 1 out]
        n197 = Multiply(x=w383, y=8.0) -> (x*y=w374:dbl)
        n198 = Increment(x=w374) -> (x+1=w373:dbl)
        "x*y" <- w373
        n199 = In Range and Coerce(upper limit=10.0, x=w373, lower limit=0.0) -> (coerced(x)=w375:dbl)  [unwired: 1 out]
        "output voltage" <- w375
        n200 = case shown="False" "Enable?" {
          tunnel: w375 -> [_ w403]
          frame False {
          }
          frame True {
            "Waveform Chart" <- w403
          }
        }
        n201 = call-poly <vilib>:"DAQmx Write.vi"("task/channels in"=w397, "data"=w375, "error in"=w396) -> ("task out"=w399:refnum<k21>, "error out"=w398:errorcluster)  [unwired: 10 in, 1 out]
      }
      frame "close" {
        n202 = Dequeue Element(queue=w432) -> (queue out=w431:refnum<queue>, error out=w430:errorcluster)  [unwired: 2 in, 2 out]
        n203 = Unbundle By Name(w421) -> ("dev2_data"=w422:refnum<queue>)
        n204 = Release Queue(queue=w431, error in (no error)=w430) -> ()  [unwired: 1 in, 3 out]
        n205 = Flush Queue(queue=w422) -> (queue out=w423:refnum<queue>)  [unwired: 1 in, 2 out]
        n206 = Release Queue(queue=w423) -> ()  [unwired: 2 in, 3 out]
      }
      frame "release" {
        n207 = Dequeue Element(queue=w443) -> ()  [unwired: 2 in, 4 out]
        n208 = call <vilib>:"DAQmx Stop Task.vi"("task/channels in"=w440, "error in"=w439) -> ("task out"=w438:refnum<k21>, "error out"=w437:errorcluster)  [unwired: 12 in]
        n209 = call <vilib>:"DAQmx Clear Task.vi"("task in"=w438, "error in"=w437) -> ("error out"=w442:errorcluster)  [unwired: 13 in]
      }
      frame "initialize" {
        w456 = -1 items=["Default"=-1, "RSE"=10083, "Differential"=10106, "Pseudodifferential"=12529] ("output terminal configuration")
        n210 = Dequeue Element(queue=w451) -> ()  [unwired: 2 in, 4 out]
        n211 = call-poly <vilib>:"DAQmx Create Virtual Channel.vi"("maximum value"=10.0, "minimum value"=0.0, "output terminal configuration"=w456, "physical channels"="physical channels", "error in"=w459) -> ("task out"=w455:refnum<k21>, "error out"=w454:errorcluster)  [unwired: 9 in]
        n212 = call <vilib>:"DAQmx Start Task.vi"("task/channels in"=w455, "error in"=w454) -> ("task out"=w453:refnum<k21>, "error out"=w452:errorcluster)  [unwired: 12 in]
      }
    }
    "meas. velocity" <- w349
    "DAC error" <- w363
  }
